vi "symbol map im.vi"() -> ()   [LabVIEW 2014]
panel:
  out "Init Data Out":fxp<+/-,16,1>[](array[numeric])=[0.70709228515625, 0.70709228515625, 0.70709228515625, 0.70709228515625, 0.70709228515625, 0.70709228515625, 0.70709228515625, 0.70709228515625, 0.50506591796875, 0.50506591796875, 0.50506591796875, 0.50506591796875, 0.50506591796875, 0.50506591796875, 0.50506591796875, 0.50506591796875, 0.10101318359375, 0.10101318359375, 0.10101318359375, 0.10101318359375, 0.10101318359375, 0.10101318359375, 0.10101318359375, 0.10101318359375, 0.30303955078125, 0.30303955078125, 0.30303955078125, 0.30303955078125, 0.30303955078125, 0.30303955078125, 0.30303955078125, 0.30303955078125, -0.70709228515625, -0.70709228515625, -0.70709228515625, -0.70709228515625, -0.70709228515625, -0.70709228515625, -0.70709228515625, -0.70709228515625, -0.50506591796875, -0.50506591796875, -0.50506591796875, -0.50506591796875, -0.50506591796875, -0.50506591796875, -0.50506591796875, -0.50506591796875, -0.10101318359375, -0.10101318359375, -0.10101318359375, -0.10101318359375, -0.10101318359375, -0.10101318359375, -0.10101318359375, -0.10101318359375, -0.30303955078125, -0.30303955078125, -0.30303955078125, -0.30303955078125, -0.30303955078125, -0.30303955078125, -0.30303955078125, -0.30303955078125]
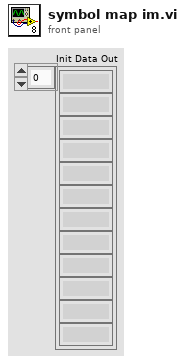
[diagram p1: front panel]
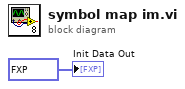
[diagram p0: block diagram]
diagram:
  "Init Data Out" <- fxp<+/-,16,1>[] [0.70709228515625, 0.70709228515625, 0.70709228515625, 0.70709228515625, 0.70709228515625, 0.70709228515625, 0.70709228515625, 0.70709228515625, 0.50506591796875, 0.50506591796875, 0.50506591796875, 0.50506591796875, 0.50506591796875, 0.50506591796875, 0.50506591796875, 0.50506591796875, 0.10101318359375, 0.10101318359375, 0.10101318359375, 0.10101318359375, 0.10101318359375, 0.10101318359375, 0.10101318359375, 0.10101318359375, 0.30303955078125, 0.30303955078125, 0.30303955078125, 0.30303955078125, 0.30303955078125, 0.30303955078125, 0.30303955078125, 0.30303955078125, -0.70709228515625, -0.70709228515625, -0.70709228515625, -0.70709228515625, -0.70709228515625, -0.70709228515625, -0.70709228515625, -0.70709228515625, -0.50506591796875, -0.50506591796875, -0.50506591796875, -0.50506591796875, -0.50506591796875, -0.50506591796875, -0.50506591796875, -0.50506591796875, -0.10101318359375, -0.10101318359375, -0.10101318359375, -0.10101318359375, -0.10101318359375, -0.10101318359375, -0.10101318359375, -0.10101318359375, -0.30303955078125, -0.30303955078125, -0.30303955078125, -0.30303955078125, -0.30303955078125, -0.30303955078125, -0.30303955078125, -0.30303955078125] ("im")
